vi "Compare Arrays.vi"(2 "OSC Configuration Control":T1(array[cluster])=[[{"Signal Type"=enum."Sine Wave", "DC"=0.0, "Amplitude"=0.001, "frequency"=2.0, "Phase"=0.0}, {"Signal Type"=enum."Sine Wave", "DC"=0.0, "Amplitude"=0.0, "frequency"=2.0, "Phase"=0.0}, {"Signal Type"=enum."Sine Wave", "DC"=0.0, "Amplitude"=0.0, "frequency"=20.0, "Phase"=0.0}], [{"Signal Type"=enum."Sine Wave", "DC"=0.0, "Amplitude"=0.0, "frequency"=2.0, "Phase"=0.0}, {"Signal Type"=enum."Sine Wave", "DC"=0.0, "Amplitude"=0.0, "frequency"=2.0, "Phase"=0.0}, {"Signal Type"=enum."Sine Wave", "DC"=0.0, "Amplitude"=0.0, "frequency"=20.0, "Phase"=0.0}]] {"frequency" step=0.001 format="%.3p"; "Amplitude" format="%0.2p"; "DC" min=-0.99 max=0.99 format="%.2p"}, 3 "OSC Global Variable":T1(array[cluster])=[[{"Signal Type"=enum."Sine Wave", "DC"=0.0, "Amplitude"=0.001, "frequency"=2.0, "Phase"=0.0}, {"Signal Type"=enum."Sine Wave", "DC"=0.0, "Amplitude"=0.0, "frequency"=2.0, "Phase"=0.0}, {"Signal Type"=enum."Sine Wave", "DC"=0.0, "Amplitude"=0.0, "frequency"=20.0, "Phase"=0.0}], [{"Signal Type"=enum."Sine Wave", "DC"=0.0, "Amplitude"=0.0, "frequency"=2.0, "Phase"=0.0}, {"Signal Type"=enum."Sine Wave", "DC"=0.0, "Amplitude"=0.0, "frequency"=2.0, "Phase"=0.0}, {"Signal Type"=enum."Sine Wave", "DC"=0.0, "Amplitude"=0.0, "frequency"=20.0, "Phase"=0.0}]] {"frequency" step=0.001 format="%.3p"; "Amplitude" format="%0.2p"; "DC" min=-0.99 max=0.99 format="%.2p"}) -> (0 "all the same?":bool, 1 "OSC Global Variable output":T1(array[cluster]))   [LabVIEW 2013, in "Lock-In Variable Channels_2.lvclass"]
uses:
  Lock-In Variable Channels_2.lvclass
panel:
  out "number of columns":i32
  out "number of rows":i32
  in  "index column":i32=1
  out "index row":i32=1
  out "appended array":bool[](array[boolean])
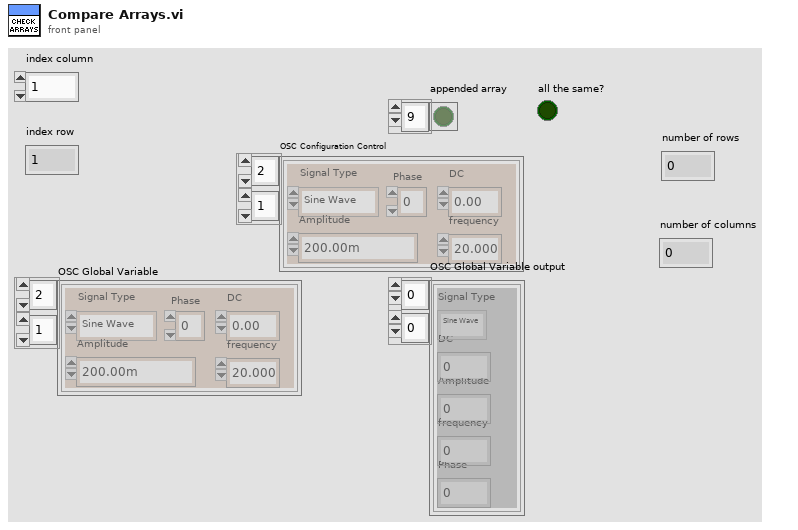
[diagram p1: front panel]
types:
  T1 = cluster{"Signal Type":enum16{"Sine Wave", "Triangle Wave", "Square Wave", "Sawtooth Wave"}, "DC":dbl, "Amplitude":dbl, "frequency":dbl, "Phase":dbl}[][]
  T2 = cluster{"Signal Type":u16, "DC":dbl, "Amplitude":dbl, "frequency":dbl, "Phase":dbl}[][]
  T3 = cluster{"Signal Type":u16, "DC":dbl, "Amplitude":dbl, "frequency":dbl, "Phase":dbl}[]
  T4 = cluster{"Signal Type":u16, "DC":dbl, "Amplitude":dbl, "frequency":dbl, "Phase":dbl}
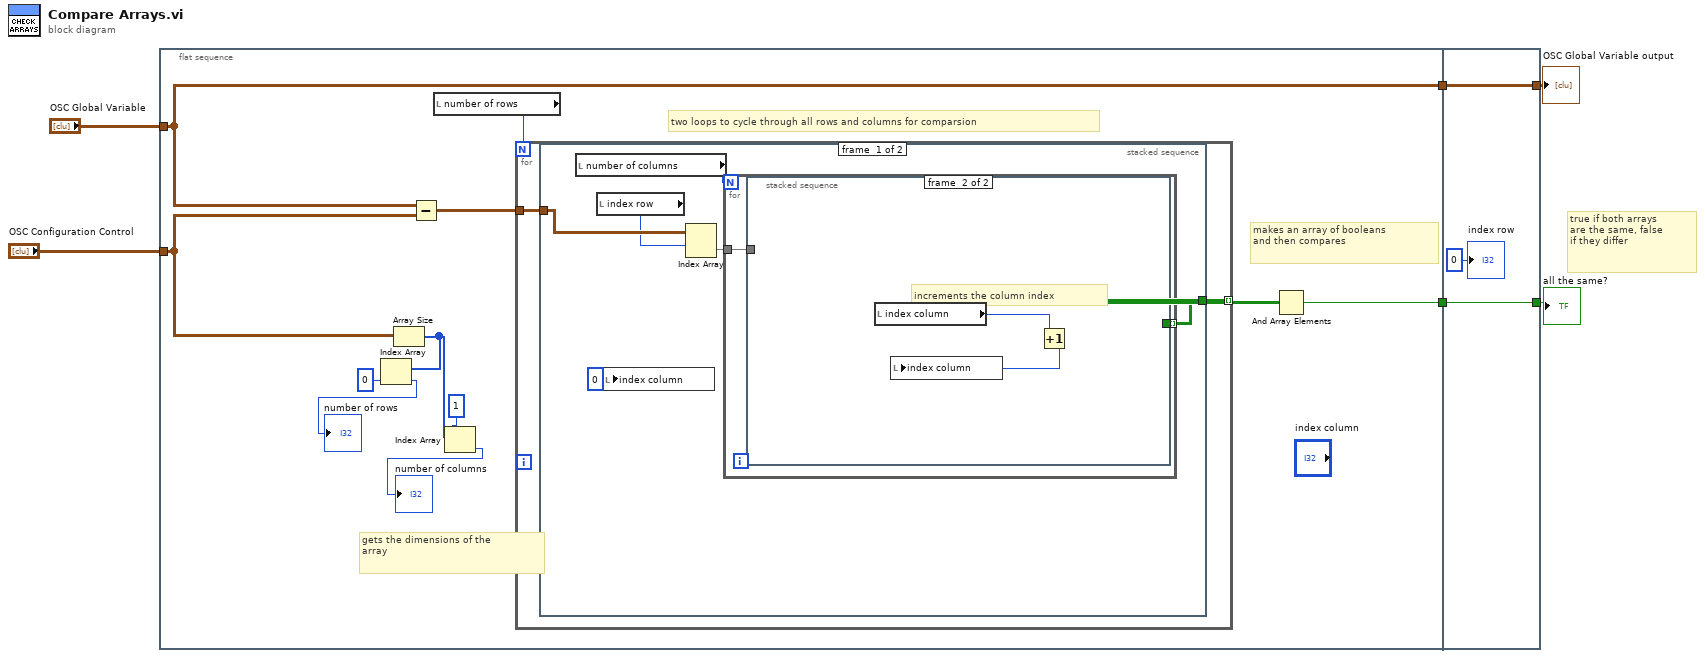
[diagram p0: block diagram]
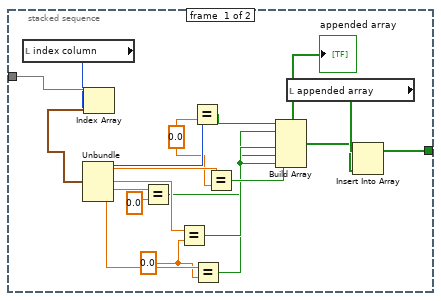
[diagram p2: hidden frame]
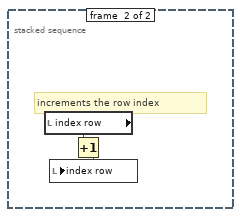
[diagram p3: hidden frame]
diagram:
  # "true if both arrays\nare the same, false\nif they differ"
  n1 = flat-sequence {
    tunnel: [w9] -> w5
    tunnel: "OSC Global Variable" -> [w8]
    tunnel: [w8] -> w3
    tunnel: "OSC Configuration Control" -> [w7]
    tunnel: [w52] -> w6
    tunnel: w5 -> [w52]
    tunnel: w3 -> [w51]
    tunnel: [w51] -> w2
    frame #0 {
      # "gets the dimensions of the \narray"
      # "two loops to cycle through all rows and columns for comparsion"
      # "makes an array of booleans\nand then compares"
      n2 = Array Size(array=w7) -> (size(s)=w12:i32[])
      n3 = Index Array(array=w12, index=0) -> (element=→"number of rows":i32)
      n4 = Subtract(x=w8, y=w7) -> (x-y=w17:T2)
      n5 = local read "number of rows"() -> (w16:i32)
      n6 = Index Array(array=w12, index=1) -> (element=→"number of columns":i32)
      n7 = for {
        N: w16 -> [_]
        tunnel: w17 -> [w19]
        tunnel: [w18] -> w15 mode=indexing
        n8 = stacked-sequence {
          tunnel: w19 -> [w25 _]
          tunnel: [w23 _] -> w18
          frame #0 {
            n9 = local read "number of columns"() -> (w21:i32)
            n10 = local read "index row"() -> (w24:i32)
            n11 = local write "index column"(0 ("index column")) -> ()
            n12 = Index Array(array=w25, index (row)=w24) -> (element=w22:T3)  [unwired: 1 in]
            n13 = for {
              N: w21 -> [_]
              tunnel: [w27] -> w23 mode=indexing
              tunnel: w22 -> [w26]
              n14 = stacked-sequence {
                tunnel: [w31 _] -> w27
                tunnel: w26 -> [w30 _]
                frame #0 {
                  w35 = 0.0 ("y")
                  w40 = 0.0 ("y")
                  n15 = local read "index column"() -> (w28:i32)
                  n16 = Index Array(array=w30, index=w28) -> (element=w29:T4)
                  n17 = Unbundle(w29) -> ("Signal Type"=w44:u16, "DC"=w43:dbl, "Amplitude"=w42:dbl, "frequency"=w45:dbl, "Phase"=w41:dbl)
                  n18 = Equal?(x=w45, y=0.0) -> (x = y?=w36:bool)
                  n19 = Equal?(x=w42, y=w40) -> (x = y?=w38:bool)
                  n20 = Equal?(x=w44, y=w35) -> (x = y?=w34:bool)
                  n21 = Equal?(x=w41, y=w40) -> (x = y?=w37:bool)
                  n22 = Equal?(x=w43, y=w35) -> (x = y?=w39:bool)
                  n23 = Build Array(w34, w36, w39, w38, w37, w36) -> (w32:bool[])
                  "appended array" <- w32
                  n24 = local read "appended array"() -> (w33:bool[])
                  n25 = Insert Into Array(array=w33, new element=w32) -> (w31:bool[])  [unwired: 1 in]
                }
                frame #1 {
                  # "increments the column index"
                  n26 = local read "index column"() -> (w48:i32)
                  n27 = Increment(x=w48) -> (x+1=w47:i32)
                  n28 = local write "index column"(w47) -> ()
                }
              }
            }
          }
          frame #1 {
            # "increments the row index"
            n29 = local read "index row"() -> (w50:i32)
            n30 = Increment(x=w50) -> (x+1=w49:i32)
            n31 = local write "index row"(w49) -> ()
          }
        }
      }
      n32 = And Array Elements(Boolean array=w15) -> (logical AND=w9:bool)
    }
    frame #1 {
      "index row" <- 0 ("index row")
    }
  }
  "all the same?" <- w6
  "OSC Global Variable output" <- w2
